vi "Init Bfr Tx - Data.vi"(7 "Data Access":refnum<class "Data Access Engine.lvclass">, 8 "error in (no error)":errorcluster, 11 "Parameters":variant) -> (0 "error out":errorcluster, 3 "Tx Loop Data":T1 {"Data Buffer" format="%016x"})   [LabVIEW 2016, in "UDP-Custom-Device Engine.lvlib"]
uses:
  UDP-Custom-Device Engine.lvlib
  <vilib>/NI/NIVS Inline Async API/_Data Access Engine/Data Access Engine/Data Access Engine.lvclass
  Types/Engine - Buffered Tx Loop Data.ctl
  Shared/Types/Shared - Header Details.ctl
  Shared/Types/Shared - Buffered.PacketInfo.ctl
  Shared/Types/Shared - Pointer Encoding.ctl
  <vilib>/NI/NIVS Inline Async API/_Data Access Engine/Data Access Engine/Types/ReadWrite.DVR.ctl
  <vilib>/NI/NIVS Inline Async API/_Data Access Engine/Access Type Classes/ReadWrite/ReadWrite.lvclass
  <vilib>/NI/NIVS Inline Async API/_Data Access Engine/Data Access Engine/Types/Read.DVR.ctl
  <vilib>/NI/NIVS Inline Async API/_Data Access Engine/Access Type Classes/Read/Read.lvclass
  <vilib>/NI/NIVS Inline Async API/_Data Access Engine/Data Access Engine/Types/Write.DVR.ctl
  <vilib>/NI/NIVS Inline Async API/_Data Access Engine/Access Type Classes/Write/Write.lvclass
  Shared/Types/Shared - Duplex Settings.ctl
  Shared/Types/Shared - Tx.PacketInfo.ctl
  Shared/Types/Shared - Channel Data Type.ctl
  <vilib>/NI/NIVS Inline Async API/_Data Access Engine/Data Access Engine/Methods/ReadWrite.Lookup.vi
  <vilib>/NI/NIVS Inline Async API/_Data Access Engine/Data Access Engine/Methods/Read.Lookup.vi
  <vilib>/NI/NIVS Inline Async API/_Data Access Engine/Data Access Engine/Methods/Write.Lookup.vi
  Shared/UDP-Custom-Device Shared.lvlib
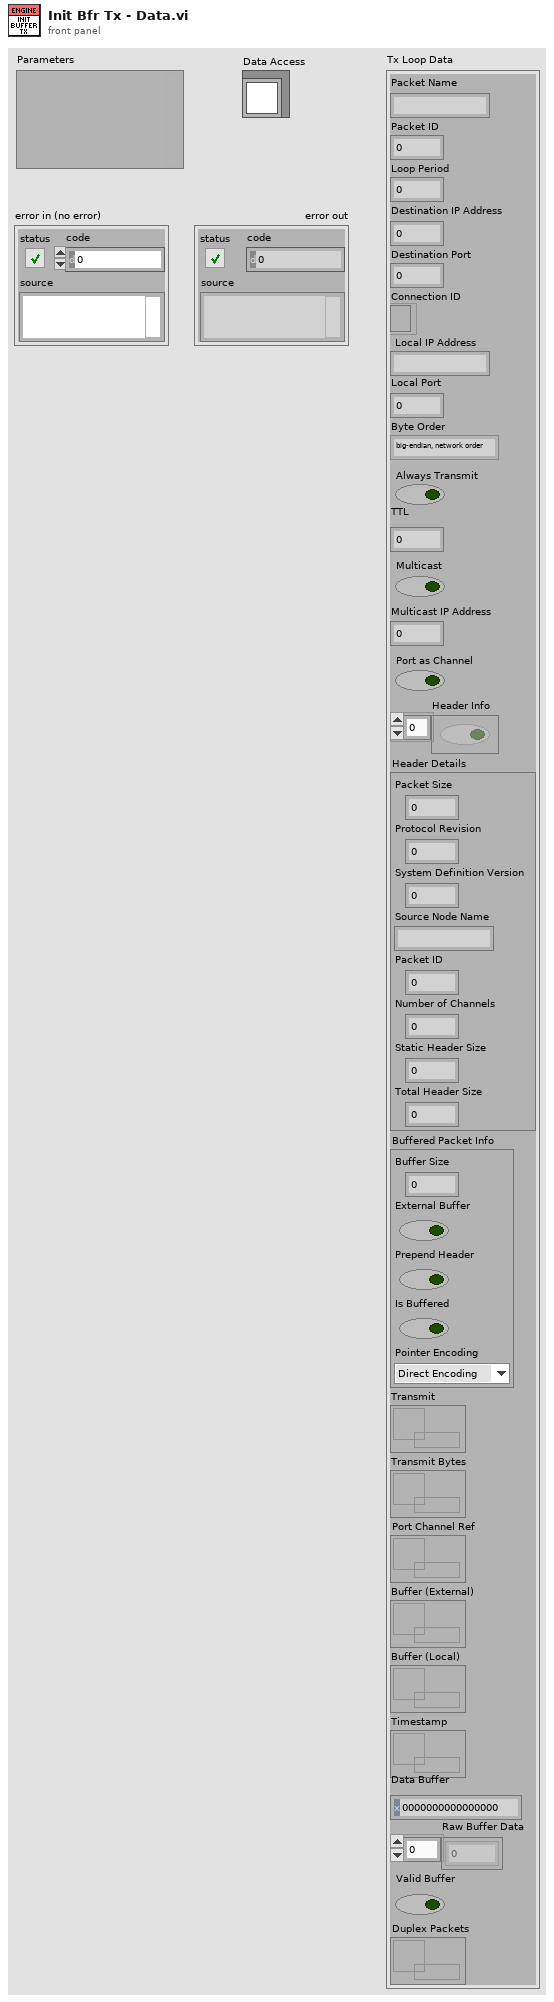
[diagram p1: front panel]
types:
  T1 = typedef "UDP-Custom-Device Engine.lvlib/Engine - Buffered Tx Loop Data.ctl" = cluster{"Packet Name":string, "Packet ID":i32, "Loop Period":u32, "Destination IP Address":u32, "Destination Port":u16, "Connection ID":refnum<k16>, "Local IP Address":string, "Local Port":i32, "Byte Order":enum16{"big-endian, network order", "native, host order", "little-endian"}, "Always Transmit":bool, "TTL":u16, "Multicast":bool, "Multicast IP Address":u32, "Port as Channel":bool, "Header Info":bool[], "Header Details":T2, "Buffered Packet Info":T3, "Transmit":T5, "Transmit Bytes":T6, "Port Channel Ref":T6, "Buffer (External)":T6, "Buffer (Local)":T7, "Timestamp":T6, "Data Buffer":u64, "Raw Buffer Data":u8[], "Valid Buffer":bool, "Duplex Packets":refnum<data-value>}
  T2 = typedef "UDP-Custom-Device Shared.lvlib/Shared - Header Details.ctl" = cluster{"Packet Size":u16, "Protocol Revision":u8, "System Definition Version":u64, "Source Node Name":string, "Packet ID":u32, "Number of Channels":u32, "Static Header Size":u16, "Total Header Size":u16}
  T3 = typedef "UDP-Custom-Device Shared.lvlib/Shared - Buffered.PacketInfo.ctl" = cluster{"Buffer Size":i32, "External Buffer":bool, "Prepend Header":bool, "Is Buffered":bool, "Pointer Encoding":T4}
  T4 = typedef "UDP-Custom-Device Shared.lvlib/Shared - Pointer Encoding.ctl" = enum16{"Direct Encoding", "Conversion Encoding"}
  T5 = typedef "Data Access Engine.lvlib/Data Access Engine.lvclass/ReadWrite.DVR.ctl" = refnum<data-value>
  T6 = typedef "Data Access Engine.lvlib/Data Access Engine.lvclass/Read.DVR.ctl" = refnum<data-value>
  T7 = typedef "Data Access Engine.lvlib/Data Access Engine.lvclass/Write.DVR.ctl" = refnum<data-value>
  T8 = typedef "UDP-Custom-Device Shared.lvlib/Shared - Tx.PacketInfo.ctl" = cluster{"Packet Name":string, "Packet ID":i32, "Decimation":u16, "Destination IP Address":string, "Destination Port":u16, "Local IP Address":string, "Local Port":u16, "Endianness":u16, "Always Transmit":bool, "TTL":u16, "Multicast":bool, "Multicast IP Address":string, "Port as Channel":bool, "Header Info":bool[], "PCL Period":u32, "Channel Data Types":T9[], "Header Details":T2, "Buffered Packet Info":T3, "Duplex Packets":refnum<data-value>}
  T9 = typedef "UDP-Custom-Device Shared.lvlib/Shared - Channel Data Type.ctl" = enum16{"Boolean", "Single", "Double", "I8", "I16", "I32", "I64", "U8", "U16", "U32", "U64"}
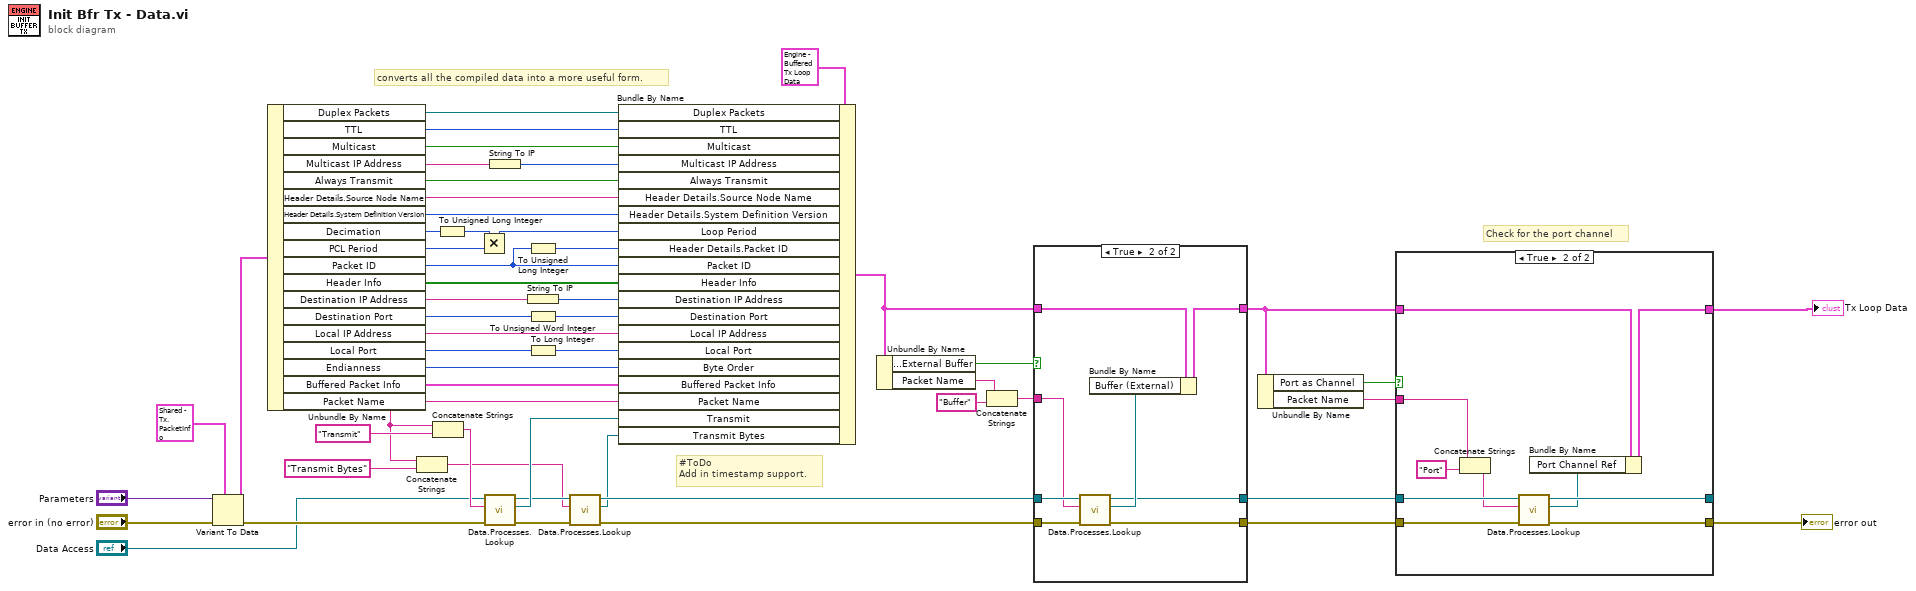
[diagram p0: block diagram]
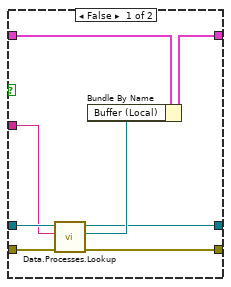
[diagram p3: hidden frame]
diagram:
  # "Check for the port channel"
  # "converts all the compiled data into a more useful form."
  # "#ToDo\nAdd in timestamp support."
  n1 = Variant To Data(error in="error in (no error)", type=T8 {"Packet Name"="", "Packet ID"=0, "Decimation"=0, "Destination IP Address"="", "Destination Port"=0, "Local IP Address"="", "Local Port"=0, "Endianness"=0, "Always Transmit"=FALSE, "TTL"=0, "Multicast"=FALSE, "Multicast IP Address"="", "Port as Channel"=FALSE, "Header Info"=[], "PCL Period"=0, "Channel Data Types"=[], "Header Details"={"Packet Size"=0, "Protocol Revision"=0, "System Definition Version"=0, "Source Node Name"="", "Packet ID"=0, "Number of Channels"=0, "Static Header Size"=0, "Total Header Size"=0}, "Buffered Packet Info"={"Buffer Size"=0, "External Buffer"=FALSE, "Prepend Header"=FALSE, "Is Buffered"=FALSE, "Pointer Encoding"=enum."Direct Encoding"}, "Duplex Packets"=refnum} ("Packet Info"), Variant="Parameters") -> (data=w51:T8, error out=w30:errorcluster)
  n2 = Unbundle By Name(w51) -> ("Duplex Packets"=w8:refnum<data-value>, "TTL"=w17:u16, "Multicast"=w18:bool, "Multicast IP Address"=w20:string, "Always Transmit"=w21:bool, "Header Details.Source Node Name"=w49:string, "Header Details.System Definition Version"=w48:u64, "Decimation"=w46:u16, "PCL Period"=w45:u32, "Packet ID"=w42:i32, "Header Info"=w41:bool[], "Destination IP Address"=w23:string, "Destination Port"=w40:u16, "Local IP Address"=w39:string, "Local Port"=w36:u16, "Endianness"=w38:u16, "Buffered Packet Info"=w34:T3, "Packet Name"=w12:string)
  n3 = Concatenate Strings(w12, "Transmit Bytes" ("Item GUID")) -> (w10:string)
  n4 = Concatenate Strings(w12, "Transmit" ("Item GUID")) -> (w31:string)
  n5 = To Unsigned Long Integer(number=w46) -> (unsigned 32bit integer=w47:u32)
  n6 = Multiply(x=w47, y=w45) -> (x*y=w44:u32)
  n7 = call-poly <vilib>:"Data.Processes.Lookup.vi"("error in (no error)"=w30, "Name"=w31, "Data Access API in"="Data Access") -> ("error out"=w14:errorcluster, "Ref"=w22:T5, "Data Access API out"=w16:refnum<class "Data Access Engine.lvclass">)  [unwired: 5 in, 1 out]
  n8 = String To IP(1:w20) -> (0:w19:u32)
  n9 = To Unsigned Long Integer(number=w42) -> (unsigned 32bit integer=w43:u32)
  n10 = String To IP(1:w23) -> (0:w24:u32)
  n11 = To Unsigned Word Integer(number=w40) -> (unsigned 16bit integer=w37:u16)
  n12 = To Long Integer(number=w36) -> (32bit integer=w35:i32)
  n13 = call-poly <vilib>:"Data.Processes.Lookup.vi"("error in (no error)"=w14, "Name"=w10, "Data Access API in"=w16) -> ("error out"=w13:errorcluster, "Ref"=w9:T6, "Data Access API out"=w15:refnum<class "Data Access Engine.lvclass">)  [unwired: 5 in, 1 out]
  n14 = Bundle By Name(cluster=T1 {"Packet Name"="", "Packet ID"=0, "Loop Period"=0, "Destination IP Address"=0, "Destination Port"=0, "Connection ID"=refnum, "Local IP Address"="", "Local Port"=0, "Byte Order"=enum."big-endian, network order", "Always Transmit"=FALSE, "TTL"=0, "Multicast"=FALSE, "Multicast IP Address"=0, "Port as Channel"=FALSE, "Header Info"=[], "Header Details"={"Packet Size"=0, "Protocol Revision"=0, "System Definition Version"=0, "Source Node Name"="", "Packet ID"=0, "Number of Channels"=0, "Static Header Size"=0, "Total Header Size"=0}, "Buffered Packet Info"={"Buffer Size"=0, "External Buffer"=FALSE, "Prepend Header"=FALSE, "Is Buffered"=FALSE, "Pointer Encoding"=enum."Direct Encoding"}, "Transmit"=refnum, "Transmit Bytes"=refnum, "Port Channel Ref"=refnum, "Buffer (External)"=refnum, "Buffer (Local)"=refnum, "Timestamp"=refnum, "Data Buffer"=0, "Raw Buffer Data"=[], "Valid Buffer"=FALSE, "Duplex Packets"=refnum} ("Tx Loop Data"), "Duplex Packets"=w8, "TTL"=w17, "Multicast"=w18, "Multicast IP Address"=w19, "Always Transmit"=w21, "Header Details.Source Node Name"=w49, "Header Details.System Definition Version"=w48, "Loop Period"=w44, "Header Details.Packet ID"=w43, "Packet ID"=w42, "Header Info"=w41, "Destination IP Address"=w24, "Destination Port"=w37, "Local IP Address"=w39, "Local Port"=w35, "Byte Order"=w38, "Buffered Packet Info"=w34, "Packet Name"=w12, "Transmit"=w22, "Transmit Bytes"=w9) -> (w27:T1)
  n15 = Unbundle By Name(w27) -> ("Buffered Packet Info.External Buffer"=w28:bool, "Packet Name"=w26:string)
  n16 = Concatenate Strings(w26, "Buffer" ("Item GUID")) -> (w25:string)
  n17 = case shown="True" w28 {
    tunnel: [w58 w66] -> w6
    tunnel: w27 -> [w59 w67]
    tunnel: [w56 w64] -> w4
    tunnel: w13 -> [w57 w65]
    tunnel: w15 -> [w62 w70]
    tunnel: w25 -> [w61 w69]
    tunnel: [w55 w63] -> w2
    frame False {
      n18 = call-poly <vilib>:"Data.Processes.Lookup.vi"("error in (no error)"=w57, "Name"=w61, "Data Access API in"=w62) -> ("error out"=w56:errorcluster, "Ref"=w60:T7, "Data Access API out"=w55:refnum<class "Data Access Engine.lvclass">)  [unwired: 5 in, 1 out]
      n19 = Bundle By Name(cluster=w59, "Buffer (Local)"=w60) -> (w58:T1)
    }
    frame True {
      n20 = call-poly <vilib>:"Data.Processes.Lookup.vi"("error in (no error)"=w65, "Name"=w69, "Data Access API in"=w70) -> ("error out"=w64:errorcluster, "Ref"=w68:T6, "Data Access API out"=w63:refnum<class "Data Access Engine.lvclass">)  [unwired: 5 in, 1 out]
      n21 = Bundle By Name(cluster=w67, "Buffer (External)"=w68) -> (w66:T1)
    }
  }
  n22 = Unbundle By Name(w6) -> ("Port as Channel"=w7:bool, "Packet Name"=w1:string)
  n23 = case shown="True" w7 {
    tunnel: w1 -> [_ w82]
    tunnel: w2 -> [w72 w81]
    tunnel: [w72 w80] -> _
    tunnel: w4 -> [w71 w79]
    tunnel: [w71 w78] -> w3
    tunnel: w6 -> [w73 w77]
    tunnel: [w73 w74] -> w5
    frame False {
    }
    frame True {
      n24 = Concatenate Strings(w82, "Port" ("Item GUID")) -> (w75:string)
      n25 = call-poly <vilib>:"Data.Processes.Lookup.vi"("error in (no error)"=w79, "Name"=w75, "Data Access API in"=w81) -> ("error out"=w78:errorcluster, "Ref"=w76:T6, "Data Access API out"=w80:refnum<class "Data Access Engine.lvclass">)  [unwired: 5 in, 1 out]
      n26 = Bundle By Name(cluster=w77, "Port Channel Ref"=w76) -> (w74:T1)
    }
  }
  "Tx Loop Data" <- w5
  "error out" <- w3
